vi "peak - fit phase around center.vi"(5 "Phase":dbl[](array[numeric]), 6 "main VI  path":path, 7 "omega":dbl[](array[numeric]), 8 "weights":dbl[](array[numeric]), 9 "guess at theta":dbl, 10 "guess at gamma":dbl, 11 "guess at omega":dbl) -> (1 "fit for theta":dbl, 2 "fit for gamma":dbl, 3 "fit for omega":dbl)   [LabVIEW 2021]
uses:
  <vilib>/gmath/NumericalOptimization/LM model function reference.ctl
  <vilib>/gmath/NumericalOptimization/Nonlinear Curve Fit LM.vi
  <vilib>/gmath/NI_Gmath.lvlib
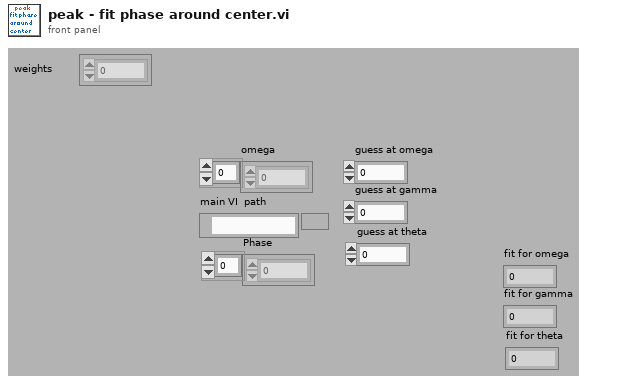
[diagram p1: front panel]
types:
  T1 = typedef "NI_Gmath.lvlib/LM model function reference.ctl" = refnum<vi>
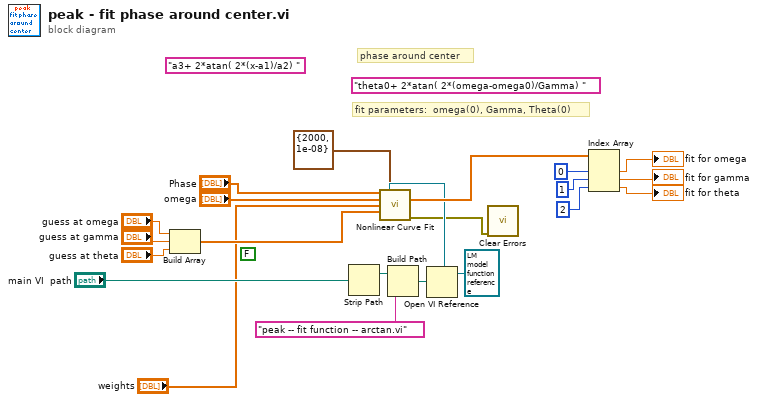
[diagram p0: block diagram]
diagram:
  (unwired) "a3+ 2*atan( 2*(x-a1)/a2) " ("model")
  (unwired) FALSE
  (unwired) "theta0+ 2*atan( 2*(omega-omega0)/Gamma) " ("model")
  # "phase around center"
  # "fit parameters:  omega(0), Gamma, Theta(0)"
  n1 = Build Array("guess at omega", "guess at gamma", "guess at theta") -> (w13:dbl[])
  n2 = Strip Path(path="main VI  path") -> (stripped path=w7:path)  [unwired: 1 out]
  n3 = Build Path(base path=w7, name or relative path="peak -- fit function -- arctan.vi" ("f(x,a) VI name Complex")) -> (appended path=w5:path)
  n4 = Open VI Reference(type specifier VI Refnum (for type only)=T1 refnum ("f(x,a)"), vi path=w5) -> (vi reference=w4:T1)  [unwired: 1 in, 4 out]
  n5 = call-poly <vilib>:"Nonlinear Curve Fit.vi"("Y"="Phase", "f(x,a)"=w4, "X"="omega", "Weight"="weights", "initial parameters"=w13, "termination"=cluster{"max iteration":i32, "tolerance":dbl} {"max iteration"=2000, "tolerance"=1e-08}) -> ("best fit parameters"=w12:dbl[], "error out"=w2:errorcluster)  [unwired: 4 in, 4 out]
  n6 = call <vilib>:"Clear Errors.vi"("error in (no error)"=w2) -> ()  [unwired: 5 in, 2 out]
  n7 = Index Array(array=w12, index #1=0, index #2=1, index #3=2) -> (element #1=→"fit for omega":dbl, element #2=→"fit for gamma":dbl, element #3=→"fit for theta":dbl)
